vi "Esophageal_Generate_Image_Filename.vi"(9 "Image Number":i32, 10 "HRME Gain":u32, 11 "HRME Exposure":u32) -> (2 "Notification Text":string, 3 "Image Filename":string)   [LabVIEW 2021]
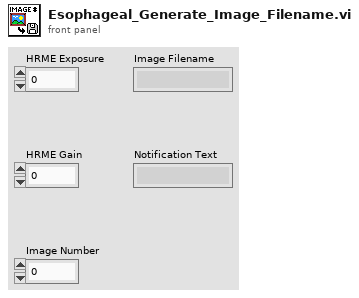
[diagram p1: front panel]
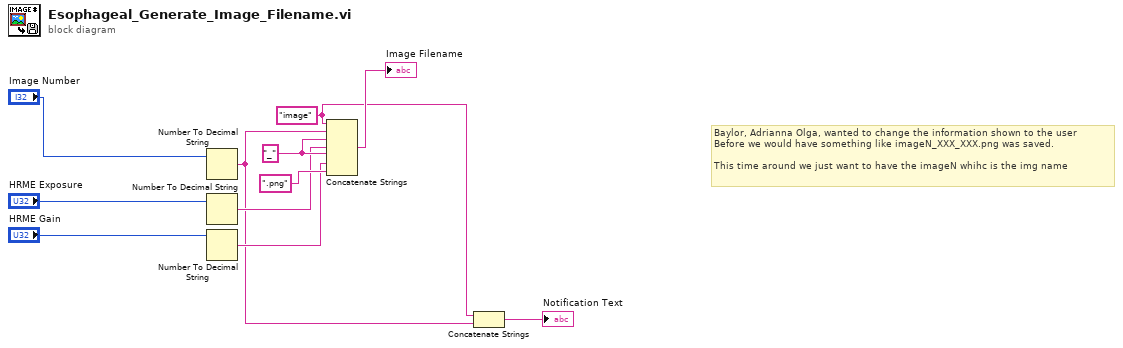
[diagram p0: block diagram]
diagram:
  w2 = "image" ("string")
  w7 = "_" ("string")
  # "Baylor, Adrianna Olga, wanted to change the information shown to the user\nBefore we would have something like imageN_XXX_XXX.png was saved.\n\nThis time around we just want to have the imageN whihc is the img name"
  n1 = Number To Decimal String(number="Image Number") -> (decimal integer string=w3:string)  [unwired: 1 in]
  n2 = Number To Decimal String(number="HRME Exposure") -> (decimal integer string=w6:string)  [unwired: 1 in]
  n3 = Number To Decimal String(number="HRME Gain") -> (decimal integer string=w8:string)  [unwired: 1 in]
  n4 = Concatenate Strings(w2, w3, w7, w6, w7, w8, ".png" ("string")) -> (→"Image Filename":string)
  n5 = Concatenate Strings(w2, w3) -> (→"Notification Text":string)
